vi "Get Error Message.vi"(8 "Error In":errorcluster) -> (0 "Error Out":errorcluster, 1 "Call Chain":string[](array[string]), 4 "Time Stamp":timestamp, 6 "Error Source":string, 7 "Error Message":string)   [LabVIEW 2016, in "Stream Error.lvlib"]
doc: "--\nCopyright © 2017 Composed SystemsI All rights reserved.\n\nAuthor: Jon McBee <jon.mcbee@composed.io>\n\nThis library is provided \"AS IS\" ,WITHOUT WARRANTIES OR\nCONDITIONS OF ANY KIND, either express or implied.\n\nComposed Systems -- composed.io\n\nStream 0.0.1.1\nJon McBee - Composed Systems\nCopyright (c) 2017, Composed Systems"
uses:
  <userlib>/Composed Systems/Stream/Error/Stream Error.lvlib
  <userlib>/Composed Systems/Stream/Error/Classes/Error Interface/Error UID.ctl
  <userlib>/Composed Systems/Stream/Error/Classes/Error Interface/Error Interface.lvclass
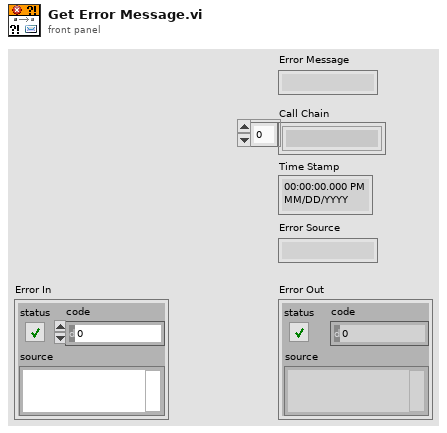
[diagram p1: front panel]
types:
  T1 = typedef "Stream Error.lvlib/Error Interface.lvclass/Error UID.ctl" = u16
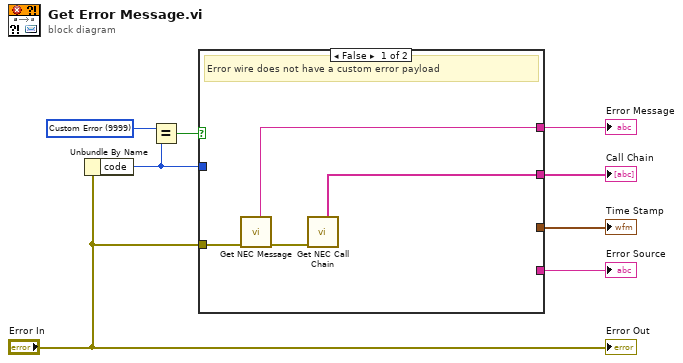
[diagram p0: block diagram]
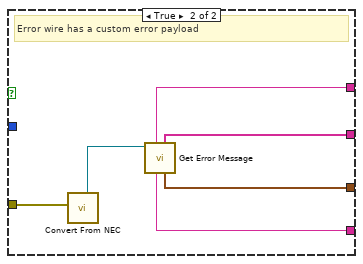
[diagram p2: hidden frame]
diagram:
  w5 = T1 9999 items=["Custom Error"=9999] ("Custom Error Codes")
  n1 = Unbundle By Name("Error In") -> ("code"=w7:i32)
  n2 = Equal?(x=w5, y=w7) -> (x = y?=w8:bool)
  n3 = case shown="False" w8 {
    tunnel: w7 -> [_ _]
    tunnel: [w12 w13] -> w1
    tunnel: [w9 w14] -> w6
    tunnel: "Error In" -> [w11 w18]
    tunnel: [_ w16] -> w3
    tunnel: [_ w15] -> w2
    frame False {
      # "Error wire does not have a custom error payload"
      n4 = call <userlib>:"Get NEC Message.vi"("error in (no error)"=w11) -> ("error out"=w10:errorcluster, "Message"=w9:string)  [unwired: 9 in]
      n5 = call <userlib>:"Get NEC Call Chain.vi"("error in (no error)"=w10) -> ("Call Chain"=w12:string[])  [unwired: 9 in, 1 out]
    }
    frame True {
      # "Error wire has a custom error payload"
      n6 = call <userlib>:"Convert From NEC.vi"("error in (no error)"=w18) -> ("Error Interface out"=w17:refnum<class "Error Interface.lvclass">)  [unwired: 9 in, 1 out]
      n7 = call-dynamic "Get Error Message.vi"("Error Interface in"=w17) -> ("Time Stamp"=w15:timestamp, "Call Chain"=w13:string[], "Error Source"=w16:string, "Error Message"=w14:string)  [unwired: 6 in, 1 out]
    }
  }
  "Error Message" <- w6
  "Error Source" <- w3
  "Time Stamp" <- w2
  "Call Chain" <- w1
  "Error Out" <- "Error In"
